vi "GrabCallBackThread1.vi"(11 "Error IN":errorcluster) -> (15 "Error OUT":errorcluster)   [LabVIEW 2014]
uses:
  <vilib>/addons/PixeLINK/Low Level Functions/TRANSLATION.llb/TDPU-Translation-CallBackFlags.ctl
  <vilib>/addons/PixeLINK/Low Level Functions/TRANSLATION.llb/TDPU-Translation-CallbacksInfo.ctl
  <vilib>/addons/PixeLINK/Low Level Functions/ACQUISITION.llb/TDPU-Acquisition-Frame_Desc.ctl
  <vilib>/addons/PixeLINK/Low Level Functions/TRANSLATION.llb/TDPU-Translation-PixelFormat.ctl
  PxLLabVIEW.dll
panel:
  out "Intensity Graph":u16[][](graph)
  out "Frame Number":u32
  out "Missed Frames":u32
  out "PixelAddressingValue.fValue":dbl format="%.2f"
  out "ROI.fHeight":dbl format="%.2f"
  out "ROI.fWidth":dbl format="%.2f"
  out "FrameData_FORMAT":T1 items=["PIXEL_FORMAT_MONO8", "PIXEL_FORMAT_MONO16", "PIXEL_FORMAT_YUV422", "PIXEL_FORMAT_BAYER8", "PIXEL_FORMAT_BAYER16", "PIXEL_FORMAT_RGB24", "PIXEL_FORMAT_RGB48"]
  out "FRAME_DESC":T2 {"PixelAddressingMode"."fValue" format="%.2f"; "Rotate"."fValue" format="%.2f"; "WhiteShading"."fBlueGain" format="%.2f"; "WhiteShading"."fGreenGain" format="%.2f"; "WhiteShading"."fRedGain" format="%.2f"; "AutoROI"."fHeight" format="%.2f"; "AutoROI"."fWidth" format="%.2f"; "AutoROI"."fTop" format="%.2f"; "AutoROI"."fLeft" format="%.2f"; "ExtendedShutter"."fKneePoint" format="%.2f"; "PixelFormat"."fValue" format="%.2f"; "PixelAddressingValue"."fValue" format="%.2f"; "Flip"."fVertical" format="%.2f"; "Flip"."fHorizontal" format="%.2f"; "ROI"."fHeight" format="%.2f"; "ROI"."fWidth" format="%.2f"; "ROI"."fTop" format="%.2f"; "ROI"."fLeft" format="%.2f"; "FrameRate"."fValue" format="%.2f"; "GPIO"."fParameter3" format="%.2f"; "GPIO"."fParameter2" format="%.2f"; "GPIO"."fParameter1" format="%.2f"; "GPIO"."fPolarity" format="%.2f"; "GPIO"."fMode" format="%.2f"; "OpticalFilter"."fValue" format="%.2f"; "Tilt"."fValue" format="%.2f"; "Pan"."fValue" format="%.2f"; "Zoom"."fValue" format="%.2f"; "Trigger"."fParameter" format="%.2f"; "Trigger"."fDelay" format="%.2f"; "Trigger"."fPolarity" format="%.2f"; "Trigger"."fType" format="%.2f"; "Trigger"."fMode" format="%.2f"; "Temperature"."fValue" format="%.2f"; "Focus"."fValue" format="%.2f"; "Iris"."fValue" format="%.2f"; "Gain"."fValue" format="%.2f"; "Shutter"."fValue" format="%.2f"; "Gamma"."fValue" format="%.2f"; "Saturation"."fValue" format="%.2f"; "Hue"."fValue" format="%.2f"; "WhiteBalance"."fValue" format="%.2f"; "Sharpness"."fValue" format="%.2f"; "AutoExposure"."fValue" format="%.2f"; "Brightness"."fValue" format="%.2f"; "fFrameTime" format="%.2f"}
  in  "CallbacksInfo IN":T3 {"uOverlayUse" items=["OVERLAY_PREVIEW             0x01", "OVERLAY_FORMAT_IMAGE  0x02", "OVERLAY_FORMAT_CLIP     0x04", "OVERLAY_FRAME                 0x08"]}
  out "FrameData":u8[](array[numeric]) format="%.0x"
  in  "Path IN":path
  in  "hCamera IN":u32
  in  "uOverlayUse IN":T4 items=["OVERLAY_PREVIEW             0x01", "OVERLAY_FORMAT_IMAGE  0x02", "OVERLAY_FORMAT_CLIP     0x04", "OVERLAY_FRAME                 0x08"]
  in  "Occurrence IN":refnum<k4>
  in  "Stop":bool
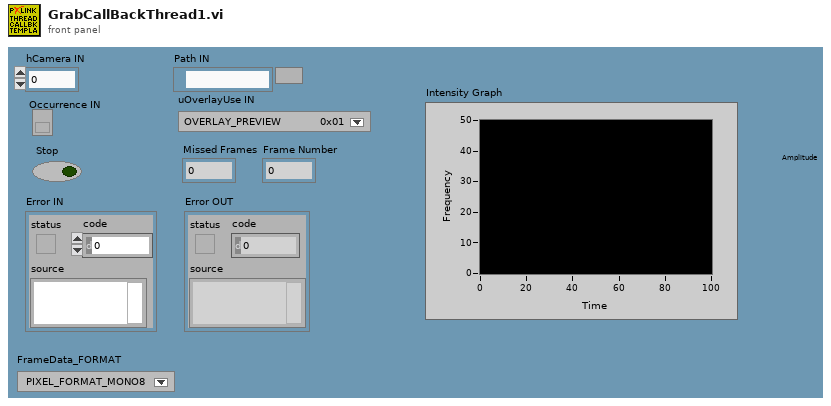
[diagram p1: front panel]
types:
  T1 = typedef "TDPU-Translation-PixelFormat.ctl" = u32
  T2 = typedef "TDPU-Acquisition-Frame_Desc.ctl" = cluster{"uSize":u32, "fFrameTime":dbl, "uFrameNumber":u32, "Brightness":cluster{"fValue":dbl}, "AutoExposure":cluster{"fValue":dbl}, "Sharpness":cluster{"fValue":dbl}, "WhiteBalance":cluster{"fValue":dbl}, "Hue":cluster{"fValue":dbl}, "Saturation":cluster{"fValue":dbl}, "Gamma":cluster{"fValue":dbl}, "Shutter":cluster{"fValue":dbl}, "Gain":cluster{"fValue":dbl}, "Iris":cluster{"fValue":dbl}, "Focus":cluster{"fValue":dbl}, "Temperature":cluster{"fValue":dbl}, "Trigger":cluster{"fMode":dbl, "fType":dbl, "fPolarity":dbl, "fDelay":dbl, "fParameter":dbl}, "Zoom":cluster{"fValue":dbl}, "Pan":cluster{"fValue":dbl}, "Tilt":cluster{"fValue":dbl}, "OpticalFilter":cluster{"fValue":dbl}, "GPIO":cluster{"fMode":dbl[], "fPolarity":dbl[], "fParameter1":dbl[], "fParameter2":dbl[], "fParameter3":dbl[]}, "FrameRate":cluster{"fValue":dbl}, "ROI":cluster{"fLeft":dbl, "fTop":dbl, "fWidth":dbl, "fHeight":dbl}, "Flip":cluster{"fHorizontal":dbl, "fVertical":dbl}, "PixelAddressingValue":cluster{"fValue":dbl}, "PixelFormat":cluster{"fValue":dbl}, "ExtendedShutter":cluster{"fKneePoint":dbl[]}, "AutoROI":cluster{"fLeft":dbl, "fTop":dbl, "fWidth":dbl, "fHeight":dbl}, "WhiteShading":cluster{"fRedGain":dbl, "fGreenGain":dbl, "fBlueGain":dbl}, "Rotate":cluster{"fValue":dbl}, "PixelAddressingMode":cluster{"fValue":dbl}}
  T3 = typedef "TDPU-Translation-CallbacksInfo.ctl" = cluster{"Occurrence":refnum<k4>, "hCamera":u32, "uOverlayUse":T4, "Path":path, "bGetClip":bool, "uNumberofFrameCaptured":u32, "error (Get Clip) ":errorcluster, "TerminationOccurence":refnum<k4>, "PDS Clip Path":path, "AVI Clip Path":path}
  T4 = typedef "TDPU-Translation-CallBackFlags.ctl" = u32
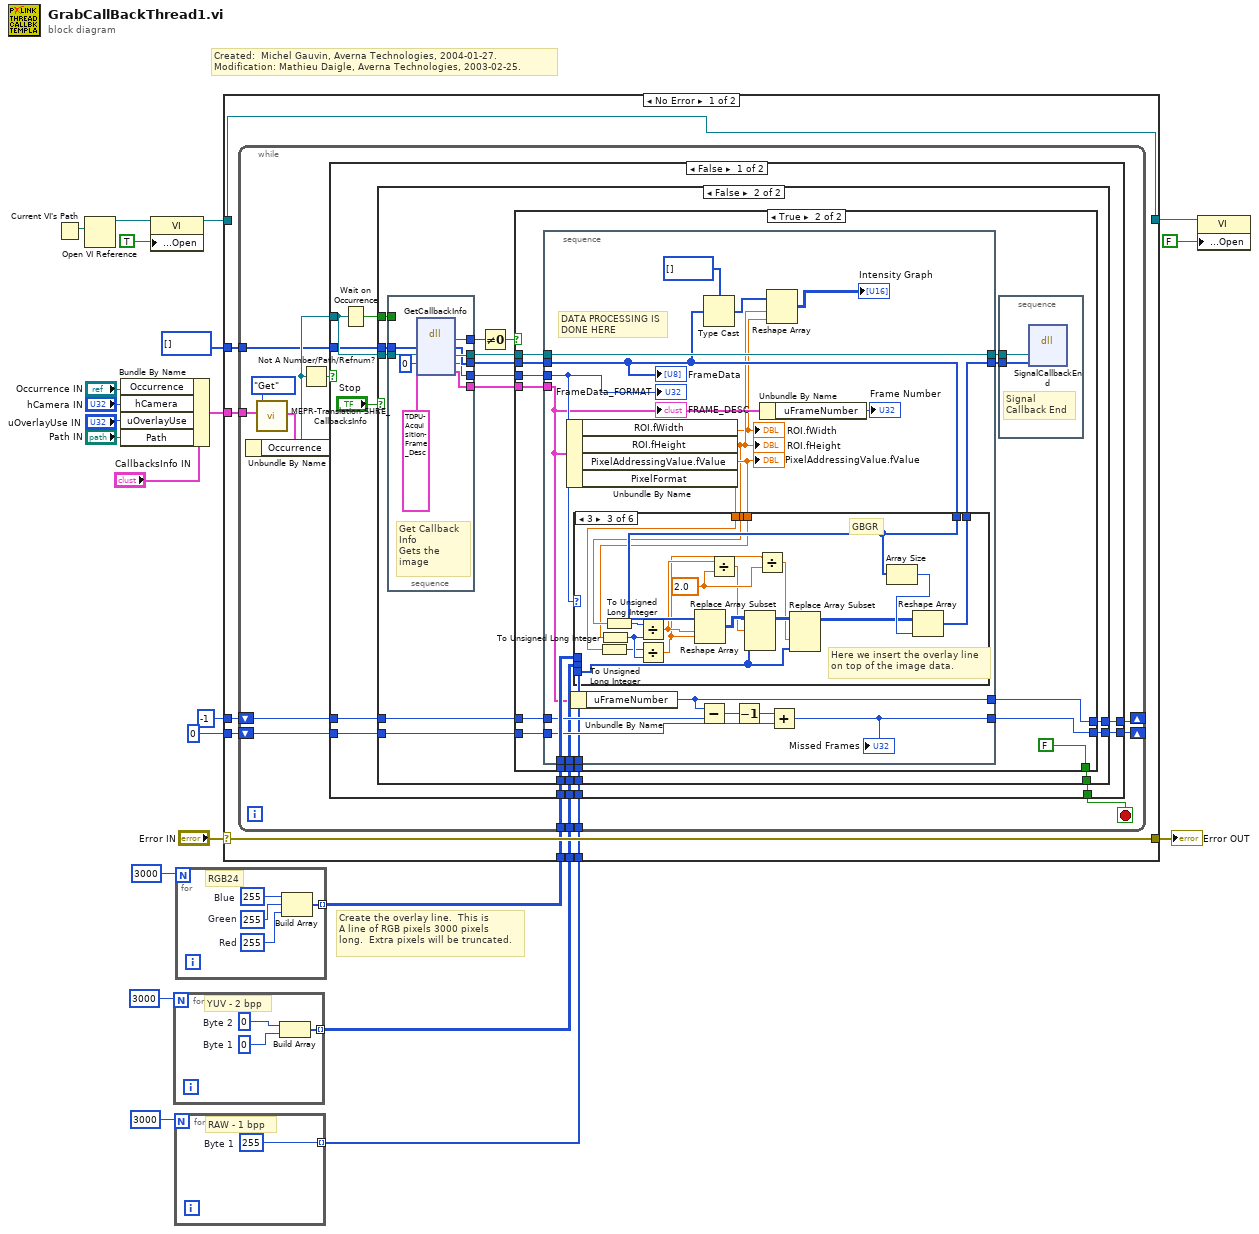
[diagram p0: block diagram]
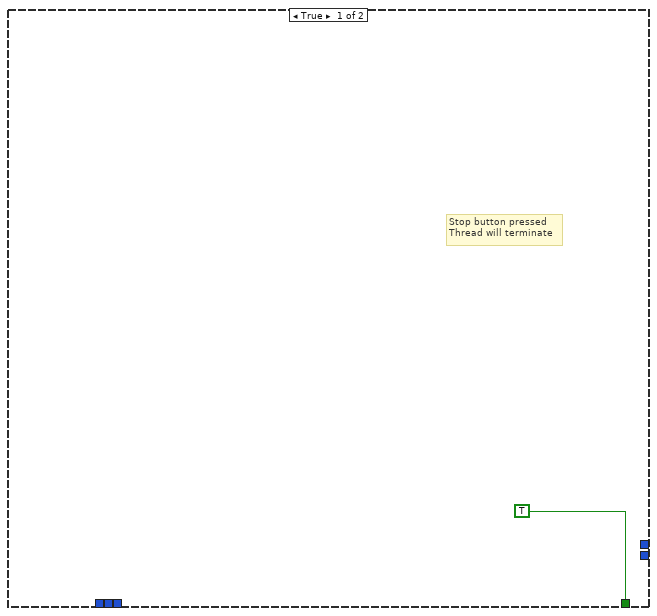
[diagram p2: hidden frame]
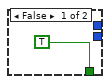
[diagram p3: hidden frame]
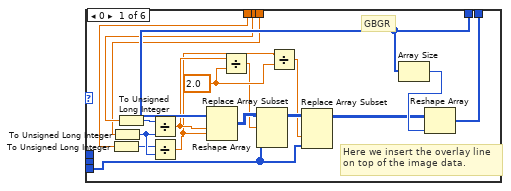
[diagram p4: hidden frame]
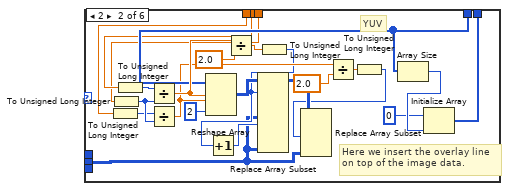
[diagram p5: hidden frame]
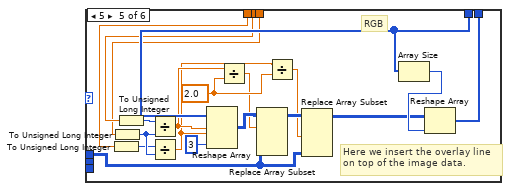
[diagram p7: hidden frame]
diagram:
  # "Create the overlay line.  This is \nA line of RGB pixels 3000 pixels\nlong.  Extra pixels will be truncated."
  # "Created:  Michel Gauvin, Averna Technologies, 2004-01-27.\nModification: Mathieu Daigle, Averna Technologies, 2003-02-25."
  n1 = Current VI's Path() -> (path=w22:path)
  n2 = Open VI Reference(vi path=w22) -> (vi reference=w21:refnum<vi>)  [unwired: 5 in, 1 out]
  n3 = Bundle By Name(cluster="CallbacksInfo IN", "Occurrence"="Occurrence IN", "hCamera"="hCamera IN", "uOverlayUse"="uOverlayUse IN", "Path"="Path IN") -> (w15:T3)
  n4 = property class="VI"(reference=w21, "Front Panel Window:Open"=TRUE) -> (reference out=w19:refnum<vi>)  [unwired: 1 in, 1 out]
  n5 = for {
    N: 3000 -> [_]
    tunnel: [w24] -> w3 mode=indexing
    w25 = u8 0  # Byte 1
    w26 = u8 0  # Byte 2
    # "YUV - 2 bpp"
    n6 = Build Array(w26, w25) -> (w24:u8[])
  }
  n7 = for {
    N: 3000 -> [_]
    tunnel: [w27] -> w1 mode=indexing
    w27 = u8 255  # Byte 1
    # "RAW - 1 bpp"
  }
  n8 = for {
    N: 3000 -> [_]
    tunnel: [w28] -> w7 mode=indexing
    w29 = u8 255  # Red
    w30 = u8 255  # Green
    w31 = u8 255  # Blue
    # "RGB24"
    n9 = Build Array(w31, w30, w29) -> (w28:u8[])
  }
  n10 = case shown="No Error" "Error IN" {
    selector: "Error IN" -> [w40 w214]
    tunnel: [w40 w214] -> w23
    tunnel: w19 -> [w39 w213]
    tunnel: [w39 w213] -> w17
    tunnel: w15 -> [w38 _]
    tunnel: u8[] [] -> [w37 _]
    tunnel: w7 -> [w36 _]
    tunnel: u32 0 -> [w35 _]
    tunnel: -1 -> [w34 _]
    tunnel: w3 -> [w33 _]
    tunnel: w1 -> [w32 _]
    frame No Error {
      n11 = while {
        tunnel: w38 -> [w52]
        tunnel: w37 -> [w48]
        tunnel: w36 -> [w47]
        shift-right: [w46] -> _
        shift-left: w34 -> [w45]
        shift-right: [w43] -> _
        shift-left: w35 -> [w44]
        tunnel: w33 -> [w42]
        tunnel: w32 -> [w41]
        stop <- w53 stop-if-true
        n12 = call <vilib>:"MEPR-Translation-SHRE_CallbacksInfo.vi"("Action"=enum16{"Get", "Clear", "Init", "Set"}."Get", "CallbackInfo IN"=w52) -> ("CallbackInfo OUT"=w51:T3)  [unwired: 15 in, 2 out]
        n13 = Unbundle By Name(w51) -> ("Occurrence"=w50:refnum<k4>)
        n14 = Not A Number/Path/Refnum?(number/path/refnum=w50) -> (NaN/Path/Refnum?=w54:bool)
        n15 = case shown="False" w54 {
          selector: w54 -> [_ w212]
          tunnel: w50 -> [w66 _]
          tunnel: [w55 w212] -> w53
          tunnel: w48 -> [w63 _]
          tunnel: w47 -> [w62 _]
          tunnel: [w61 _] -> w46
          tunnel: w45 -> [w60 _]
          tunnel: w44 -> [w59 _]
          tunnel: [w58 _] -> w43
          tunnel: w42 -> [w57 _]
          tunnel: w41 -> [w56 _]
          frame False {
            n16 = Wait on Occurrence(2:w66) -> (0:w65:bool)  [unwired: 2 in]
            n17 = case shown="False" "Stop" {
              tunnel: w66 -> [_ w84]
              tunnel: w65 -> [_ w83]
              tunnel: w63 -> [_ w80]
              tunnel: w62 -> [_ w77]
              tunnel: [_ w76] -> w61
              tunnel: w60 -> [_ w75]
              tunnel: w59 -> [_ w74]
              tunnel: [_ w73] -> w58
              tunnel: w57 -> [_ w72]
              tunnel: w56 -> [_ w71]
              tunnel: [TRUE w68] -> w55
              frame True {
                # "Stop button pressed\nThread will terminate"
              }
              frame False {
                n18 = stacked-sequence {
                  tunnel: w84 -> [w210]
                  tunnel: [w211] -> w69
                  tunnel: w83 -> [_]
                  tunnel: [w208] -> w82
                  tunnel: [w209] -> w81
                  tunnel: w80 -> [w207]
                  tunnel: [w204] -> w79
                  tunnel: [w203] -> w78
                  frame #0 {
                    # "Get Callback Info\nGets the image"
                    n19 = dll-call lib="PxLLabVIEW.dll" fn="GetCallbackInfo"("output param"=w207, "Occurrence"=w210, "pDataFormat"=u32 0, "FRAME_DESC"=T2 {"uSize"=0, "fFrameTime"=0.0, "uFrameNumber"=0, "Brightness"={"fValue"=0.0}, "AutoExposure"={"fValue"=0.0}, "Sharpness"={"fValue"=0.0}, "WhiteBalance"={"fValue"=0.0}, "Hue"={"fValue"=0.0}, "Saturation"={"fValue"=0.0}, "Gamma"={"fValue"=0.0}, "Shutter"={"fValue"=0.0}, "Gain"={"fValue"=0.0}, "Iris"={"fValue"=0.0}, "Focus"={"fValue"=0.0}, "Temperature"={"fValue"=0.0}, "Trigger"={"fMode"=0.0, "fType"=0.0, "fPolarity"=0.0, "fDelay"=0.0, "fParameter"=0.0}, "Zoom"={"fValue"=0.0}, "Pan"={"fValue"=0.0}, "Tilt"={"fValue"=0.0}, "OpticalFilter"={"fValue"=0.0}, "GPIO"={"fMode"=[], "fPolarity"=[], "fParameter1"=[], "fParameter2"=[], "fParameter3"=[]}, "FrameRate"={"fValue"=0.0}, "ROI"={"fLeft"=0.0, "fTop"=0.0, "fWidth"=0.0, "fHeight"=0.0}, "Flip"={"fHorizontal"=0.0, "fVertical"=0.0}, "PixelAddressingValue"={"fValue"=0.0}, "PixelFormat"={"fValue"=0.0}, "ExtendedShutter"={"fKneePoint"=[]}, "AutoROI"={"fLeft"=0.0, "fTop"=0.0, "fWidth"=0.0, "fHeight"=0.0}, "WhiteShading"={"fRedGain"=0.0, "fGreenGain"=0.0, "fBlueGain"=0.0}, "Rotate"={"fValue"=0.0}, "PixelAddressingMode"={"fValue"=0.0}}) -> (w211:i32, "output param"=w208:u8[], "Occurrence"=w209:refnum<k4>, "pDataFormat"=w203:u32, "FRAME_DESC"=w204:T2)  [unwired: 3 in, 2 out]
                  }
                }
                n20 = Not Equal To 0?(x=w69) -> (x != 0?=w70:bool)
                n21 = case shown="True" w70 {
                  tunnel: w82 -> [_ w98]
                  tunnel: w81 -> [_ w97]
                  tunnel: w79 -> [_ w95]
                  tunnel: w78 -> [_ w94]
                  tunnel: w77 -> [_ w93]
                  tunnel: [_ w86] -> w76
                  tunnel: w75 -> [_ w92]
                  tunnel: w74 -> [_ w91]
                  tunnel: [_ w90] -> w73
                  tunnel: w72 -> [_ w89]
                  tunnel: w71 -> [_ w88]
                  tunnel: [TRUE FALSE] -> w68
                  frame False {
                  }
                  frame True {
                    n22 = stacked-sequence {
                      tunnel: w97 -> [w122]
                      tunnel: [w122] -> w99
                      tunnel: w98 -> [w107]
                      tunnel: [w120] -> w96
                      tunnel: w95 -> [w109]
                      tunnel: w94 -> [w111]
                      tunnel: w93 -> [w119]
                      tunnel: [w118] -> w86
                      tunnel: w92 -> [w117]
                      tunnel: w91 -> [w114]
                      tunnel: [w113] -> w90
                      tunnel: w89 -> [w112]
                      tunnel: w88 -> [w110]
                      frame #0 {
                        # "DATA PROCESSING IS DONE HERE"
                        n23 = Unbundle By Name(w109) -> ("ROI.fWidth"=w102:dbl, "ROI.fHeight"=w103:dbl, "PixelAddressingValue.fValue"=w121:dbl)  [unwired: 1 out]
                        "ROI.fWidth" <- w102
                        "ROI.fHeight" <- w103
                        "PixelAddressingValue.fValue" <- w121
                        n24 = Unbundle By Name(w109) -> ("uFrameNumber"=w118:u32)
                        n25 = case shown="3" w111 {
                          tunnel: w103 -> [w133 w152 w174 _ w193 _]
                          tunnel: w102 -> [w129 w148 w170 _ w189 _]
                          tunnel: w121 -> [w132 w151 w173 _ w192 _]
                          tunnel: w107 -> [w138 w158 w179 w182 w198 w202]
                          tunnel: [w137 w157 w178 w182 w197 w202] -> w120
                          tunnel: w119 -> [_ _ _ _ w188 _]
                          tunnel: w112 -> [_ w142 _ _ _ _]
                          tunnel: w110 -> [w128 _ w169 _ _ _]
                          frame 0 {
                            w127 = 2.0 ("y")
                            # "GBGR"
                            # "Here we insert the overlay line\non top of the image data."
                            n26 = To Unsigned Long Integer(number=w129) -> (unsigned 32bit integer=w130:u32)
                            n27 = To Unsigned Long Integer(number=w132) -> (unsigned 32bit integer=w131:u32)
                            n28 = To Unsigned Long Integer(number=w133) -> (unsigned 32bit integer=w134:u32)
                            n29 = Divide(x=w134, y=w131) -> (x/y=w126:dbl)
                            n30 = Divide(x=w130, y=w131) -> (x/y=w125:dbl)
                            n31 = Reshape Array(w138, w126, w125) -> (w140:u8[][])
                            n32 = Divide(x=w126, y=w127) -> (x/y=w124:dbl)
                            n33 = Replace Array Subset(array=w140, new element=w128, index (row)=w124) -> (w136:u8[][])  [unwired: 1 in]
                            n34 = Divide(x=w125, y=w127) -> (x/y=w123:dbl)
                            n35 = Replace Array Subset(array=w136, new element=w128, index (col)=w123) -> (w135:u8[][])  [unwired: 1 in]
                            n36 = Array Size(array=w138) -> (size(s)=w139:i32)
                            n37 = Reshape Array(w135, w139) -> (w137:u8[])
                          }
                          frame 2 {
                            # "YUV"
                            # "Here we insert the overlay line\non top of the image data."
                            n38 = To Unsigned Long Integer(number=w148) -> (unsigned 32bit integer=w149:u32)
                            n39 = To Unsigned Long Integer(number=w151) -> (unsigned 32bit integer=w150:u32)
                            n40 = To Unsigned Long Integer(number=w152) -> (unsigned 32bit integer=w153:u32)
                            n41 = Divide(x=w153, y=w150) -> (x/y=w161:dbl)
                            n42 = Divide(x=w149, y=w150) -> (x/y=w155:dbl)
                            n43 = Reshape Array(w158, w161, w155, 2 ("dimension size")) -> (w162:u8[][][])
                            n44 = Divide(x=w161, y=2.0) -> (x/y=w147:dbl)
                            n45 = To Unsigned Long Integer(number=w147) -> (unsigned 32bit integer=w144:u32)
                            n46 = Increment(x=w144) -> (x+1=w143:u32)
                            n47 = Replace Array Subset(array=w162, new element #1=w142, index (dim 0) #1=w144, new element #2=w142, index (dim 0) #2=w143) -> (w154:u8[][][])  [unwired: 4 in]
                            n48 = Divide(x=w155, y=2.0) -> (x/y=w146:dbl)
                            n49 = To Unsigned Long Integer(number=w146) -> (unsigned 32bit integer=w145:u32)
                            n50 = Replace Array Subset(array=w154, new element=w142, index (dim 1)=w145) -> ()  [unwired: 2 in, 1 out]
                            n51 = Array Size(array=w158) -> (size(s)=w159:i32)
                            n52 = Initialize Array(u8 0, w159) -> (w157:u8[])
                          }
                          frame 3 {
                            w168 = 2.0 ("y")
                            # "GBGR"
                            # "Here we insert the overlay line\non top of the image data."
                            n53 = To Unsigned Long Integer(number=w170) -> (unsigned 32bit integer=w171:u32)
                            n54 = To Unsigned Long Integer(number=w173) -> (unsigned 32bit integer=w172:u32)
                            n55 = To Unsigned Long Integer(number=w174) -> (unsigned 32bit integer=w175:u32)
                            n56 = Divide(x=w175, y=w172) -> (x/y=w167:dbl)
                            n57 = Divide(x=w171, y=w172) -> (x/y=w166:dbl)
                            n58 = Reshape Array(w179, w167, w166) -> (w181:u8[][])
                            n59 = Divide(x=w167, y=w168) -> (x/y=w165:dbl)
                            n60 = Replace Array Subset(array=w181, new element=w169, index (row)=w165) -> (w177:u8[][])  [unwired: 1 in]
                            n61 = Divide(x=w166, y=w168) -> (x/y=w164:dbl)
                            n62 = Replace Array Subset(array=w177, new element=w169, index (col)=w164) -> (w176:u8[][])  [unwired: 1 in]
                            n63 = Array Size(array=w179) -> (size(s)=w180:i32)
                            n64 = Reshape Array(w176, w180) -> (w178:u8[])
                          }
                          frame 4 {
                          }
                          frame 5 {
                            w186 = 2.0 ("y")
                            # "RGB"
                            # "Here we insert the overlay line\non top of the image data."
                            n65 = To Unsigned Long Integer(number=w189) -> (unsigned 32bit integer=w190:u32)
                            n66 = To Unsigned Long Integer(number=w192) -> (unsigned 32bit integer=w191:u32)
                            n67 = To Unsigned Long Integer(number=w193) -> (unsigned 32bit integer=w194:u32)
                            n68 = Divide(x=w194, y=w191) -> (x/y=w187:dbl)
                            n69 = Divide(x=w190, y=w191) -> (x/y=w184:dbl)
                            n70 = Reshape Array(w198, w187, w184, 3 ("dimension size")) -> (w200:u8[][][])
                            n71 = Divide(x=w187, y=w186) -> (x/y=w185:dbl)
                            n72 = Replace Array Subset(array=w200, new element=w188, index (dim 0)=w185) -> (w196:u8[][][])  [unwired: 2 in]
                            n73 = Divide(x=w184, y=w186) -> (x/y=w183:dbl)
                            n74 = Replace Array Subset(array=w196, new element=w188, index (dim 1)=w183) -> (w195:u8[][][])  [unwired: 2 in]
                            n75 = Array Size(array=w198) -> (size(s)=w199:i32)
                            n76 = Reshape Array(w195, w199) -> (w197:u8[])
                          }
                          frame 6, Default {
                          }
                        }
                        n77 = Subtract(x=w118, y=w117) -> (x-y=w116:u32)
                        n78 = Type Cast(type=u16[] [] ("output param"), x=w107) -> (*(type *) &x=w105:u16[])
                        n79 = Decrement(x=w116) -> (x-1=w115:u32)
                        n80 = Unbundle By Name(w109) -> ("uFrameNumber"=→"Frame Number":u32)
                        n81 = Reshape Array(w105, w103, w102) -> (→"Intensity Graph":u16[][])
                        n82 = Add(x=w115, y=w114) -> (x+y=w113:u32)
                        "Missed Frames" <- w113
                        "FrameData" <- w107
                        "FRAME_DESC" <- w109
                        "FrameData_FORMAT" <- w111
                      }
                    }
                    n83 = stacked-sequence {
                      tunnel: w99 -> [w101]
                      tunnel: w96 -> [w100]
                      frame #0 {
                        # "Signal Callback End"
                        n84 = dll-call lib="PxLLabVIEW.dll" fn="SignalCallbackEnd"("Occurrence"=w101, "Data"=w100) -> ()  [unwired: 6 in, 2 out]
                      }
                    }
                  }
                }
              }
            }
          }
          frame True {
          }
        }
      }
    }
    frame Error {
    }
  }
  "Error OUT" <- w23
  n85 = property class="VI"(reference=w17, "Front Panel Window:Open"=FALSE) -> ()  [unwired: 1 in, 2 out]
